vi "Send ADC.vi"(8 "error in (no error)":errorcluster, 9 "VISA resource name":refnum<visa-resource-name>, 10 "Channel":dbl, 11 "Simulado in":refnum<class "Simulado.lvclass">) -> (0 "error out":errorcluster, 1 "VISA resource name 2":refnum<visa-resource-name>, 2 "Response":string, 3 "Simulado out":refnum<class "Simulado.lvclass">)   [LabVIEW 2020, in "Simulado.lvclass"]
uses:
  Simulado.lvclass
  Abstract/Serial Device/Serial Device.lvclass
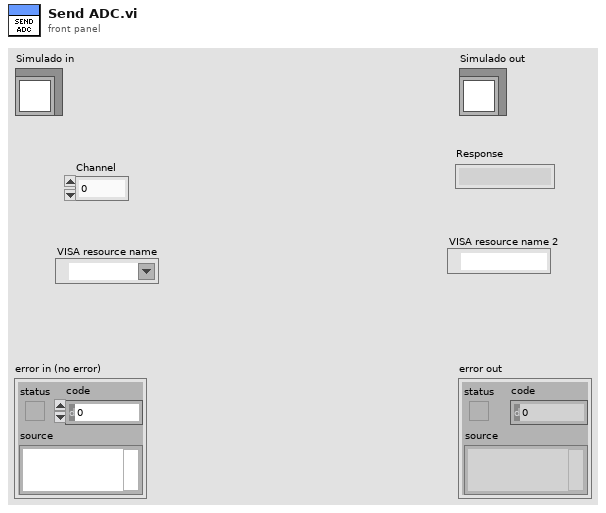
[diagram p1: front panel]
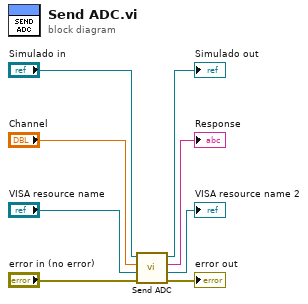
[diagram p0: block diagram]
diagram:
  n1 = call-parent "Send ADC.vi"("error in (no error)"="error in (no error)", "VISA resource name"="VISA resource name", "Channel"="Channel", "Serial Device in"="Simulado in") -> ("error out"=→"error out":errorcluster, "VISA resource name 2"=→"VISA resource name 2":refnum<visa-resource-name>, "Response"=→"Response":string, "Serial Device out"=→"Simulado out":refnum<class "Simulado.lvclass">)  [unwired: 4 in]
